vi "CalcSweepPoints.vi"(0 "Start":dbl, 5 "Stop(Use \"Span\" if it's not NaN)":dbl=nan, 7 "Step(Used if \"Points\" equals 0)":dbl, 9 "Points(0 as default)\"":i32, 11 "Span(\"Stop\" = \"Start\" + \"Span\" if not NaN)":dbl=nan, 12 "Setting":cluster{"Method":u16, "S":dbl}={"Method"=0, "S"=3.0} {"Method" items=["y=x", "y=1-(1-x)^S", "y=x^(1/S)"]}) -> (8 "SweepPoints":dbl[](array[numeric]))   [LabVIEW 2017]
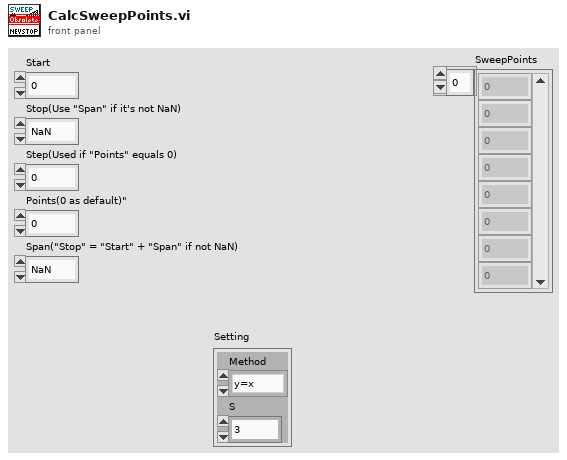
[diagram p1: front panel]
types:
  T1 = cluster{"Start":dbl, "Stop":dbl, "Step":dbl, "Points":i32, "Span":dbl}
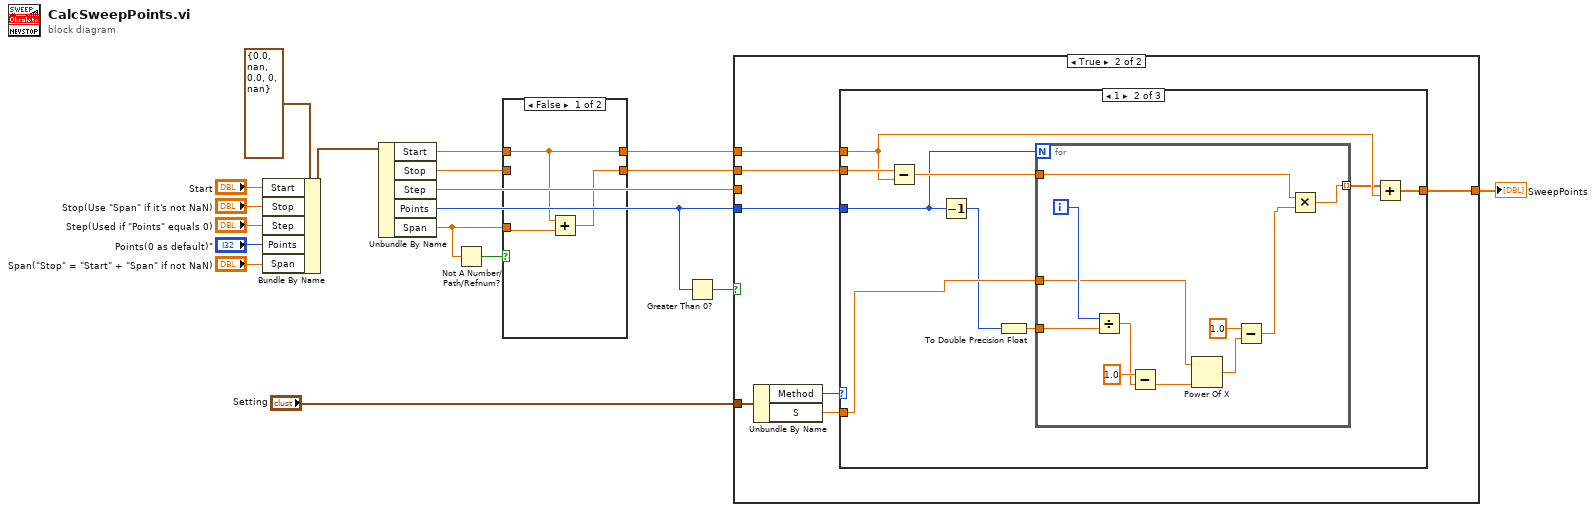
[diagram p0: block diagram]
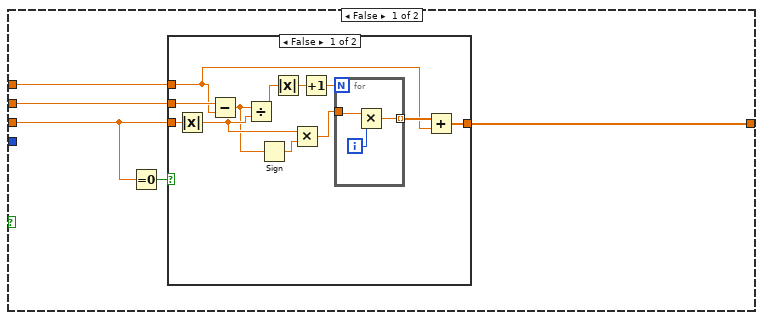
[diagram p3: hidden frame]
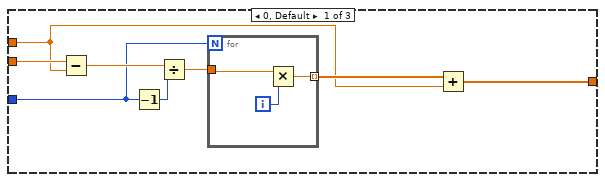
[diagram p5: hidden frame]
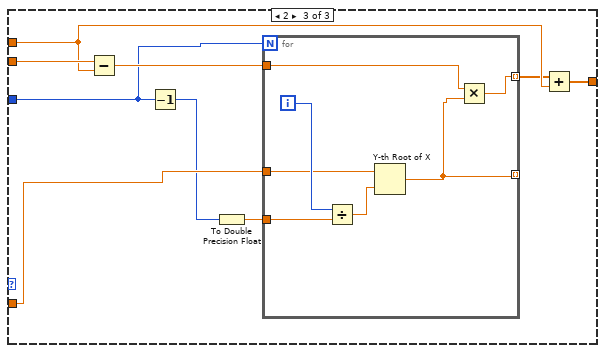
[diagram p6: hidden frame]
diagram:
  n1 = Bundle By Name(cluster=T1 {"Start"=0.0, "Stop"=nan, "Step"=0.0, "Points"=0, "Span"=nan} ("Data"), "Start"="Start", "Stop"="Stop(Use \"Span\" if it's not NaN)", "Step"="Step(Used if \"Points\" equals 0)", "Points"="Points(0 as default)\"", "Span"="Span(\"Stop\" = \"Start\" + \"Span\" if not NaN)") -> (w7:T1)
  n2 = Unbundle By Name(w7) -> ("Start"=w8:dbl, "Stop"=w10:dbl, "Step"=w18:dbl, "Points"=w17:i32, "Span"=w13:dbl)
  n3 = Not A Number/Path/Refnum?(number/path/refnum=w13) -> (NaN/Path/Refnum?=w12:bool)
  n4 = case shown="False" w12 {
    tunnel: w13 -> [w21 _]
    tunnel: [w20 w23] -> w11
    tunnel: w10 -> [_ w23]
    tunnel: [w19 w22] -> w9
    tunnel: w8 -> [w19 w22]
    frame False {
      n5 = Add(x=w19, y=w21) -> (x+y=w20:dbl)
    }
    frame True {
    }
  }
  n6 = Greater Than 0?(x=w17) -> (x > 0?=w16:bool)
  n7 = case shown="True" w16 {
    tunnel: w17 -> [_ w47]
    tunnel: w9 -> [w26 w48]
    tunnel: w11 -> [w28 w50]
    tunnel: w18 -> [w25 _]
    tunnel: [w27 w49] -> w14
    tunnel: "Setting" -> [_ w46]
    frame False {
      n8 = Equal To 0?(x=w25) -> (x = 0?=w24:bool)
      n9 = case shown="False" w24 {
        tunnel: w28 -> [w40 _]
        tunnel: [w38 _] -> w27
        tunnel: w26 -> [w37 _]
        tunnel: w25 -> [w29 _]
        frame False {
          n10 = Absolute Value(x=w29) -> (abs(x)=w33:dbl)
          n11 = Subtract(x=w40, y=w37) -> (x-y=w31:dbl)
          n12 = Divide(x=w31, y=w33) -> (x/y=w35:dbl)
          n13 = Sign(1:w31) -> (0:w30:dbl)
          n14 = Absolute Value(x=w35) -> (abs(x)=w34:dbl)
          n15 = Multiply(x=w33, y=w30) -> (x*y=w32:dbl)
          n16 = Increment(x=w34) -> (x+1=w36:dbl)
          n17 = for {
            N: w36 -> [_]
            tunnel: w32 -> [w43]
            tunnel: [w41] -> w39 mode=indexing
            i -> [w42]
            n18 = Multiply(x=w43, y=w42) -> (x*y=w41:dbl)
          }
          n19 = Add(x=w39, y=w37) -> (x+y=w38:dbl[])
        }
        frame True {
        }
      }
    }
    frame True {
      n20 = Unbundle By Name(w46) -> ("Method"=w45:u16, "S"=w44:dbl)
      n21 = case shown="1" w45 {
        tunnel: w50 -> [w58 w70 w90]
        tunnel: [w54 w67 w87] -> w49
        tunnel: w48 -> [w53 w69 w89]
        tunnel: w47 -> [w52 w62 w82]
        tunnel: w44 -> [_ w65 w85]
        frame 0, Default {
          n22 = Subtract(x=w58, y=w53) -> (x-y=w57:dbl)
          n23 = Decrement(x=w52) -> (x-1=w51:i32)
          n24 = Divide(x=w57, y=w51) -> (x/y=w56:dbl)
          n25 = for {
            N: w52 -> [_]
            tunnel: w56 -> [w61]
            tunnel: [w59] -> w55 mode=indexing
            i -> [w60]
            n26 = Multiply(x=w61, y=w60) -> (x*y=w59:dbl)
          }
          n27 = Add(x=w55, y=w53) -> (x+y=w54:dbl[])
        }
        frame 1 {
          n28 = Subtract(x=w70, y=w69) -> (x-y=w64:dbl)
          n29 = Decrement(x=w62) -> (x-1=w63:i32)
          n30 = To Double Precision Float(number=w63) -> (double precision float=w66:dbl)
          n31 = for {
            N: w62 -> [_]
            tunnel: [w79] -> w68 mode=indexing
            tunnel: w66 -> [w80]
            tunnel: w65 -> [w72]
            tunnel: w64 -> [w78]
            i -> [w81]
            n32 = Divide(x=w81, y=w80) -> (x/y=w73:dbl)
            n33 = Subtract(x=1.0, y=w73) -> (x-y=w77:dbl)
            n34 = Power Of X(1:w77, 2:w72) -> (0:w74:dbl)
            n35 = Subtract(x=1.0, y=w74) -> (x-y=w71:dbl)
            n36 = Multiply(x=w78, y=w71) -> (x*y=w79:dbl)
          }
          n37 = Add(x=w68, y=w69) -> (x+y=w67:dbl[])
        }
        frame 2 {
          n38 = Subtract(x=w90, y=w89) -> (x-y=w84:dbl)
          n39 = Decrement(x=w82) -> (x-1=w83:i32)
          n40 = To Double Precision Float(number=w83) -> (double precision float=w86:dbl)
          n41 = for {
            N: w82 -> [_]
            tunnel: [w93] -> w88 mode=indexing
            tunnel: w86 -> [w96]
            tunnel: w85 -> [w94]
            tunnel: [w92] -> _ mode=indexing
            tunnel: w84 -> [w91]
            i -> [w97]
            n42 = Divide(x=w97, y=w96) -> (x/y=w95:dbl)
            n43 = Y-th Root of X(1:w95, 2:w94) -> (0:w92:dbl)
            n44 = Multiply(x=w91, y=w92) -> (x*y=w93:dbl)
          }
          n45 = Add(x=w88, y=w89) -> (x+y=w87:dbl[])
        }
      }
    }
  }
  "SweepPoints" <- w14
